vi "isik_sayaci.vi"() -> ()   [LabVIEW 2021]
uses:
  <vilib>/Instr/_visa.llb/VISA Configure Serial Port (Instr).vi
panel:
  out "Sayaç":string
  in  "VISA resource name":refnum<visa-resource-name>
  in  "?":bool
  # "INTERFEROMETRE SAÇAK SAYACI"
  # "KÜBRA ÖZTİRYAKİ 170519031"
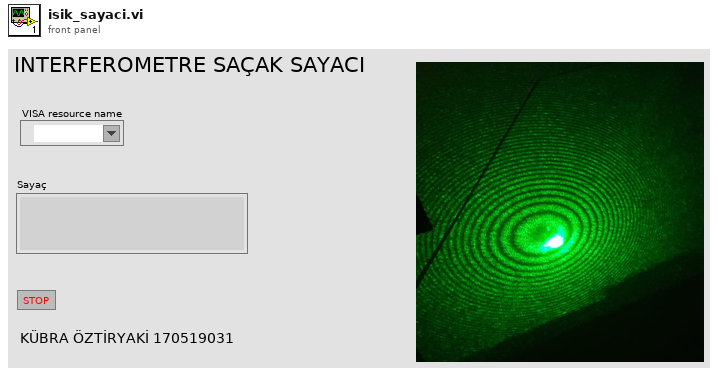
[diagram p1: front panel]
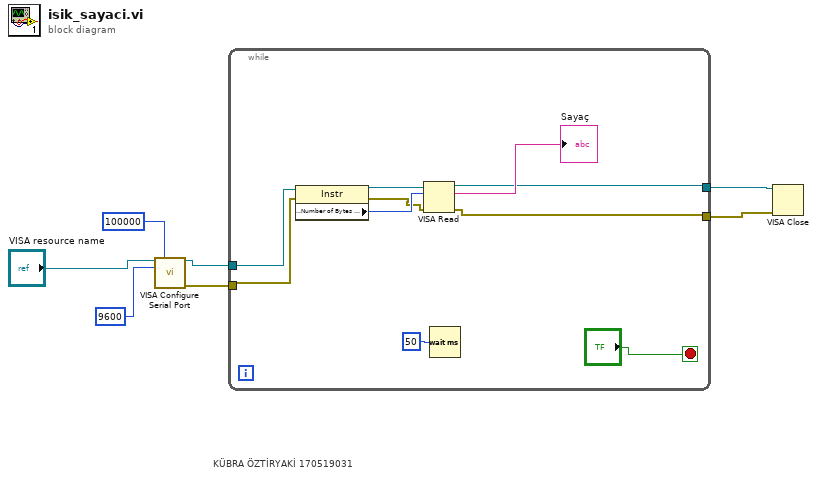
[diagram p0: block diagram]
diagram:
  # "KÜBRA ÖZTİRYAKİ 170519031"
  n1 = call-poly "VISA Configure Serial Port"("VISA resource name"="VISA resource name", "timeout (10sec)"=u32 100000, "baud rate (9600)"=u32 9600) -> ("VISA resource name out"=w4:refnum<visa-resource-name>, "error out"=w3:errorcluster)  [unwired: 11 in]
  n2 = while {
    tunnel: w4 -> [w15]
    tunnel: w3 -> [w14]
    tunnel: [w9] -> w2
    tunnel: [w8] -> w1
    stop <- "?" stop-if-true
    n3 = property class="Instr"(reference=w15, error in=w14) -> (reference out=w13:refnum<visa-resource-name>, error out=w11:errorcluster, "Serial Settings:Number of Bytes at Serial Port"=w12:u32)
    n4 = VISA Read(VISA resource name=w13, byte count=w12, error in (no error)=w11) -> (VISA resource name out=w8:refnum<visa-resource-name>, read buffer=→"Sayaç":string, error out=w9:errorcluster)  [unwired: 1 out]
    n5 = Wait (ms)(milliseconds to wait=u32 50) -> ()  [unwired: 1 out]
  }
  n6 = VISA Close(VISA resource name=w1, error in (no error)=w2) -> ()  [unwired: 1 out]
